vi "Get CITI Packages.vi"   [LabVIEW 2023, in "NI_HFNetworkAnalysis.lvlib"]
doc: "Retrieve the CITI packages available in memory for the referenced CITI file."
uses:
  NI_HFNetworkAnalysis.lvlib
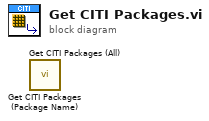
[diagram p0: block diagram]
diagram:
  n1 = call "Get CITI Packages (Package Name).vi"() -> ()  [unwired: 9 in, 3 out]
  n2 = call "Get CITI Packages (All).vi"() -> ()  [unwired: 9 in, 3 out]
